vi "运行环境动态添加删除游标（游标列表属性）.vi"() -> ()   [LabVIEW 2012]
uses:
  <vilib>/measure/NI_MABase.lvlib
panel:
  in  "删除游标":bool
  in  "添加游标":bool
  in  "游标信息":T1={"Name"="aa", "Color"=65400, "Style"=8, "Point Style"=13, "Name Visible"=TRUE, "Allow Drag"=TRUE, "Position"={"X"=0.0, "Y"=0.0}, "X Scale"=0, "Y Scale"=0, "Watch Plots"=[], "Watch All Plots"=TRUE}
  in  "停止":bool
  out "波形图":waveform(dbl)(graph)
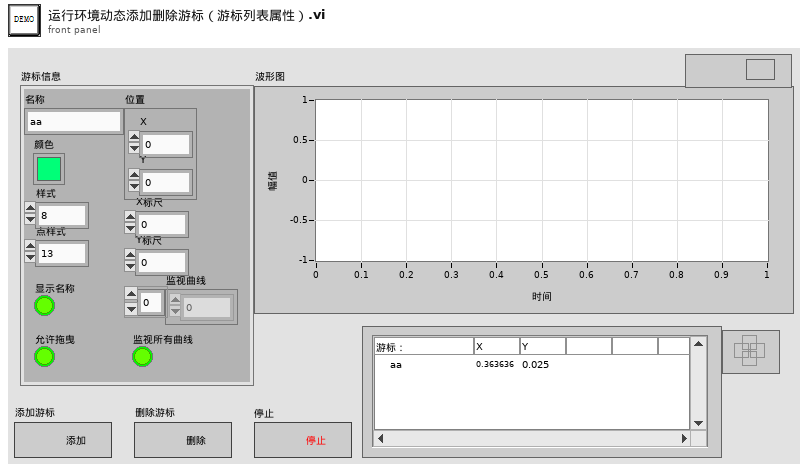
[diagram p1: front panel]
types:
  T1 = cluster{"Name":string, "Color":u32, "Style":u8, "Point Style":u8, "Name Visible":bool, "Allow Drag":bool, "Position":cluster{"X":dbl, "Y":dbl}, "X Scale":u32, "Y Scale":u32, "Watch Plots":i32[], "Watch All Plots":bool}
  T2 = cluster{"Name":string, "Color":u32, "Style":u8, "Point Style":u8, "Name Visible":bool, "Allow Drag":bool, "Cursor Mode":u32, "Plot":i32, "Index":i32, "Position":cluster{"X":dbl, "Y":dbl}, "X Scale":u32, "Y Scale":u32, "Watch Plots":i32[], "Watch All Plots":bool, "Plot Area":i32, "Label Offset":cluster{"X":dbl, "Y":dbl}}
  T3 = typedef "LVCursorListTypeDef.ctl" = cluster{"Name":string, "Color":u32, "Style":u8, "Point Style":u8, "Name Visible":bool, "Allow Drag":bool, "Cursor Mode":u32, "Plot":i32, "Index":i32, "Position":cluster{"X":dbl, "Y":dbl}, "X Scale":u32, "Y Scale":u32, "Watch Plots":i32[], "Watch All Plots":bool, "Plot Area":i32, "Label Offset":cluster{"X":dbl, "Y":dbl}}[]
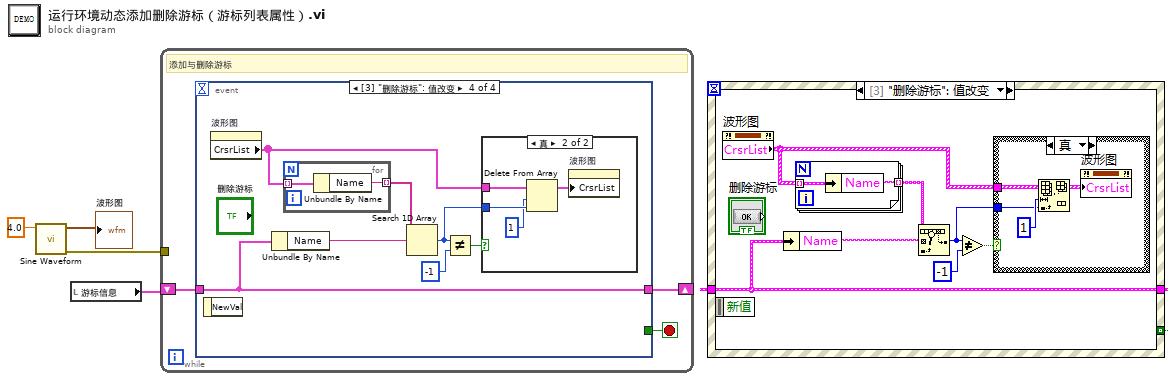
[diagram p0: block diagram]
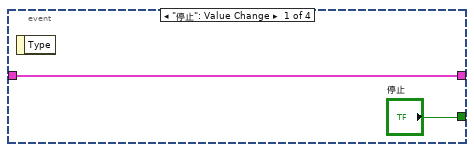
[diagram p2: hidden frame]
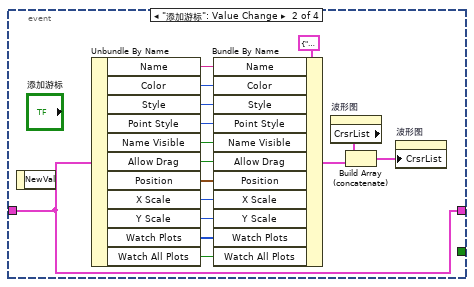
[diagram p3: hidden frame]
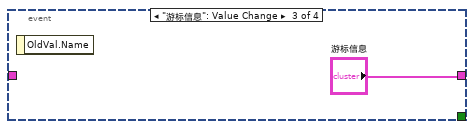
[diagram p4: hidden frame]
diagram:
  n1 = call <vilib>:"Sine Waveform.vi"("frequency"=4.0) -> ("error out"=w2:errorcluster, "signal out"=→"波形图":waveform(dbl))  [unwired: 9 in]
  n2 = local read "游标信息"() -> (w1:T1)
  n3 = while {
    tunnel: w2 -> [_]
    shift-right: [w6] -> _
    shift-left: w1 -> [w5]
    stop <- w7 stop-if-true
    # "添加与删除游标"
    n4 = event shown="[3] \"删除游标\": 值改变" {
      selector: _ -> [_ _ _ _]
      dyn-events: _ -> [_ _ _ _]
      timeout: _ -> [_ _ _ _]
      tunnel: ["停止" _ _ _] -> w7
      tunnel: [w8 w10 "游标信息" w27] -> w6
      tunnel: w5 -> [w8 w10 _ w27]
      event "停止": Value Change {
        n5 = event-data() -> ()  [unwired: 1 in, 1 out]
      }
      event "添加游标": Value Change {
        n6 = event-data() -> ()  [unwired: 1 in, 1 out]
        n7 = Unbundle By Name(w10) -> ("Name"=w24:string, "Color"=w23:u32, "Style"=w22:u8, "Point Style"=w21:u8, "Name Visible"=w20:bool, "Allow Drag"=w19:bool, "Position"=w18:cluster{"X":dbl, "Y":dbl}, "X Scale"=w17:u32, "Y Scale"=w16:u32, "Watch Plots"=w15:i32[], "Watch All Plots"=w14:bool)
        n8 = Bundle By Name(cluster=T2 {"Name"="", "Color"=0, "Style"=0, "Point Style"=0, "Name Visible"=FALSE, "Allow Drag"=FALSE, "Cursor Mode"=0, "Plot"=0, "Index"=0, "Position"={"X"=0.0, "Y"=0.0}, "X Scale"=0, "Y Scale"=0, "Watch Plots"=[], "Watch All Plots"=FALSE, "Plot Area"=0, "Label Offset"={"X"=0.0, "Y"=0.0}}, "Name"=w24, "Color"=w23, "Style"=w22, "Point Style"=w21, "Name Visible"=w20, "Allow Drag"=w19, "Position"=w18, "X Scale"=w17, "Y Scale"=w16, "Watch Plots"=w15, "Watch All Plots"=w14) -> (w12:T2)
        n9 = property on="波形图" class="WFGraph (严格)"() -> ("CrsrList"=w13:T3)  [unwired: 2 in, 2 out]
        n10 = Build Array (concatenate)(w13, w12) -> (w11:T3)
        n11 = property on="波形图" class="WFGraph (严格)"("CrsrList"=w11) -> ()  [unwired: 2 in, 2 out]
      }
      event "游标信息": Value Change {
        n12 = event-data() -> ()  [unwired: 1 in, 1 out]
      }
      event "删除游标": Value Change {
        n13 = event-data() -> ()  [unwired: 1 in, 1 out]
        n14 = property on="波形图" class="WFGraph (严格)"() -> ("CrsrList"=w29:T3)  [unwired: 2 in, 2 out]
        n15 = Unbundle By Name(w27) -> ("Name"=w32:string)
        n16 = for {
          tunnel: w29 -> [w39] mode=indexing
          tunnel: [w38] -> w33 mode=indexing
          n17 = Unbundle By Name(w39) -> ("Name"=w38:string)
        }
        n18 = Search 1D Array(1D array=w33, element=w32) -> (index of element=w28:i32)  [unwired: 1 in]
        n19 = Not Equal?(x=w28, y=-1) -> (x != y?=w31:bool)
        n20 = case shown="真" w31 {
          tunnel: w29 -> [_ w37]
          tunnel: w28 -> [_ w36]
          frame False {
          }
          frame True {
            n21 = Delete From Array(array=w37, length=1 ("长度"), index=w36) -> (array with subset deleted=w34:T3)  [unwired: 1 out]
            n22 = property on="波形图" class="WFGraph (严格)"("CrsrList"=w34) -> ()  [unwired: 2 in, 2 out]
          }
        }
      }
    }
  }
